vi "Read Frequency.vi"(8 "error in (no error)":errorcluster, 11 "Software Lock-in in":refnum<class "Software Lock-in.lvclass">) -> (0 "error out":errorcluster, 2 "Frequency":dbl, 3 "Software Lock-in out":refnum<class "Software Lock-in.lvclass">)   [LabVIEW 2015, in "Software Lock-in.lvclass"]
uses:
  Software Lock-in.lvclass
  Software Lock-in.lvclass/Software Lock-in.ctl
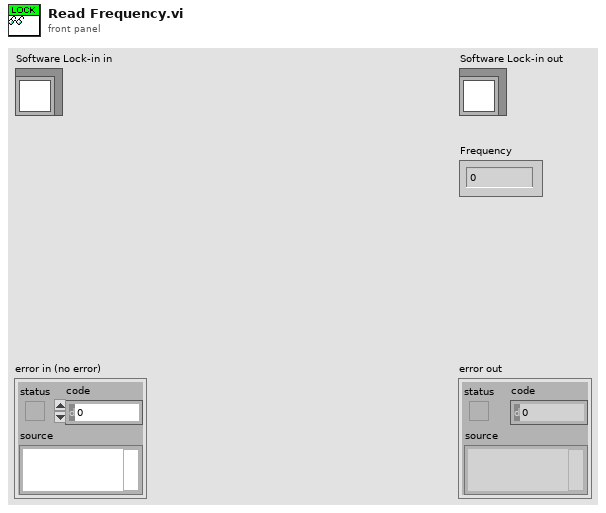
[diagram p1: front panel]
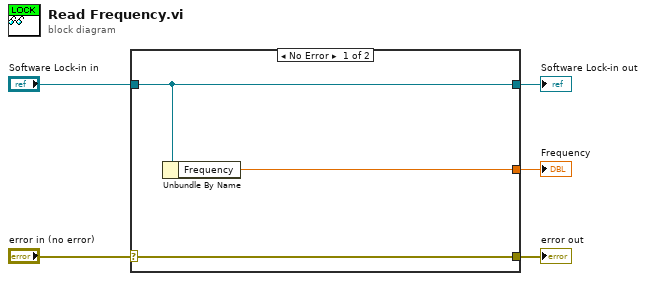
[diagram p0: block diagram]
diagram:
  n1 = case shown="No Error" "error in (no error)" {
    selector: "error in (no error)" -> [w8 w9]
    tunnel: [w8 w9] -> w4
    tunnel: [w7 w10] -> w2
    tunnel: "Software Lock-in in" -> [w7 w10]
    tunnel: [w6 _] -> w1
    frame No Error {
      n2 = Unbundle By Name(w7) -> ("Frequency"=w6:dbl)
    }
    frame Error {
    }
  }
  "error out" <- w4
  "Software Lock-in out" <- w2
  "Frequency" <- w1
